vi "Leakage_SMU_PPMU_Test.vi"(0 "Semiconductor Module Context":T4, 5 "Pin Force":T2, 7 "Pins Meas":T2[](array[typedef]), 9 "DCPower_Parameters":T1={"Output"=enum."DC Voltage", "Current_range"=0.0, "Current"=0.0, "Voltage_range"=0.0, "Voltage"=0.0, "Aperture_time"=0.0, "Source Delay"=0.0, "Sense"=1008} {"Source Delay" format="%.6p"; "Sense" items=["Local"=1008, "Remote"=1009]; "Aperture_time" format="%.6p"; "Current_range" format="%.6p"; "Current" format="%.6p"; "Voltage_range" format="%.6p"; "Voltage" format="%.6p"}, 11 "PPMU_Parameters":T3, 12 "Settling (s)":dbl format="%#_6p") -> (15 "error out":errorcluster)   [LabVIEW 2023, in "Leakage.lvlib"]
doc: "Leakage test by forcing one pin with SMU and measuring current with PPMU channels"
uses:
  Leakage.lvlib
  <vilib>/NI_TestStand_SemiconductorModule/NI_TestStand_Semiconductor_Module.lvlibp/PinMap/General/SemiconductorModuleContext.ctl
  <vilib>/NI_TestStand_SemiconductorModule/NI_TestStand_Semiconductor_Module.lvlibp/PinMap/TagProvider/TSM_Pin.ctl
  ResourceHandling/TypeDefs/RH_PPMU_Parameters.ctl
  ResourceHandling/TypeDefs/RH_DCPower_Parameters.ctl
  <instrlib>/niDigital/niDigital.llb/niDigital Output Function.ctl
  <instrlib>/niDigital/niDigital.llb/niDigital Measurement Type.ctl
  <vilib>/NI_TestStand_SemiconductorModule/NI_TestStand_Semiconductor_Module.lvlibp/PinMap/Digital Pattern/SingleSessionPinQueryContext/DigitalPatternSingleSessionPinQueryContext.lvclass
  C:/Program Files/National Instruments/LabVIEW 2023/vi.lib/NI_TestStand_SemiconductorModule/NI_TestStand_Semiconductor_Module.lvlibp/PinMap/PinQueryContext/PinQueryContext.lvclass
  <vilib>/NI_TestStand_SemiconductorModule/NI_TestStand_Semiconductor_Module.lvlibp/PinMap/Digital Pattern/PinsToNIDigitalPatternSession.vi
  <vilib>/NI_TestStand_SemiconductorModule/NI_TestStand_Semiconductor_Module.lvlibp/PinMap/DC Power/PinToNIDCPowerSessions.vi
  <vilib>/NI_TestStand_SemiconductorModule/NI_TestStand_Semiconductor_Module.lvlibp/PinMap/General/Publish/PublishDataDouble1D.vi
  <vilib>/NI_TestStand_SemiconductorModule/NI_TestStand_Semiconductor_Module.lvlibp
  ResourceHandling/ResourceHandling.lvlib
  C:/Program Files/National Instruments/LabVIEW 2023/vi.lib/NI_TestStand_SemiconductorModule/NI_TestStand_Semiconductor_Module.lvlibp/PinMap/PinQueryContext/MultiplePinSingleSessionQueryContext/MultiplePinSingleSessionQueryContext.lvclass
  C:/Program Files/National Instruments/LabVIEW 2023/vi.lib/NI_TestStand_SemiconductorModule/NI_TestStand_Semiconductor_Module.lvlibp/PinMap/Digital Pattern/SingleSessionPinQueryContext/DigitalPatternSingleSessionPinQueryContext.lvclass
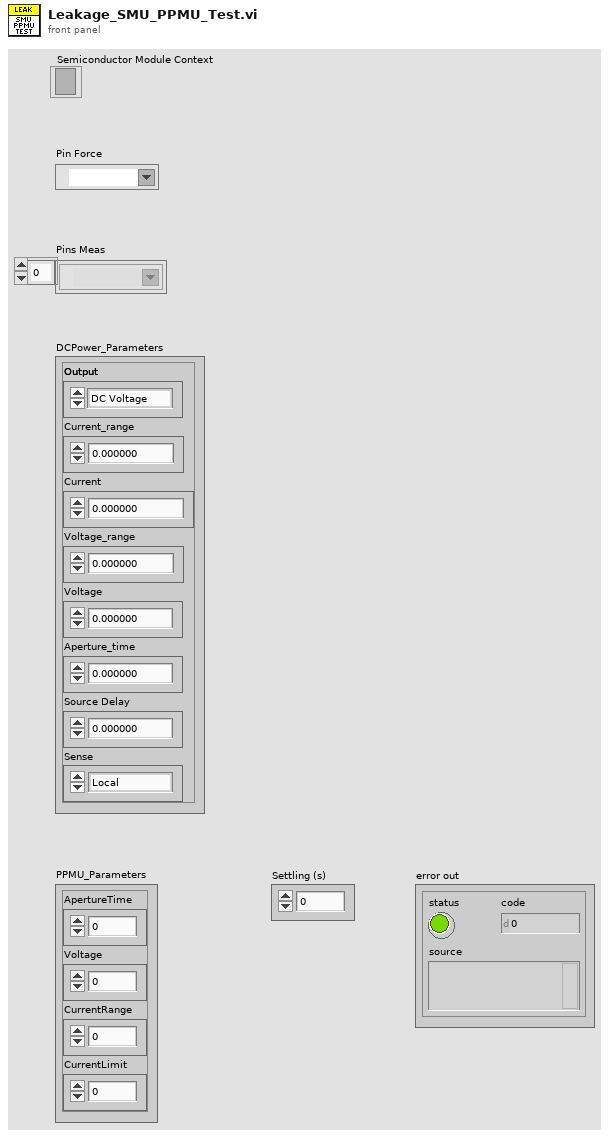
[diagram p1: front panel]
types:
  T1 = typedef "ResourceHandling.lvlib/RH_DCPower_Parameters.ctl" = cluster{"Output":enum16{"DC Voltage", "DC Current"}, "Current_range":dbl, "Current":dbl, "Voltage_range":dbl, "Voltage":dbl, "Aperture_time":dbl, "Source Delay":dbl, "Sense":i32}
  T2 = typedef "NI_TestStand_Semiconductor_Module.lvlibp/TSM_Pin.ctl" = tag
  T3 = typedef "ResourceHandling.lvlib/RH_PPMU_Parameters.ctl" = cluster{"ApertureTime":dbl, "Voltage":dbl, "CurrentRange":dbl, "CurrentLimit":dbl}
  T4 = typedef "NI_TestStand_Semiconductor_Module.lvlibp/SemiconductorModuleContext.ctl" = refnum<k7>
  T5 = typedef "niDigital Measurement Type.ctl" = i32
  T6 = typedef "niDigital Output Function.ctl" = i32
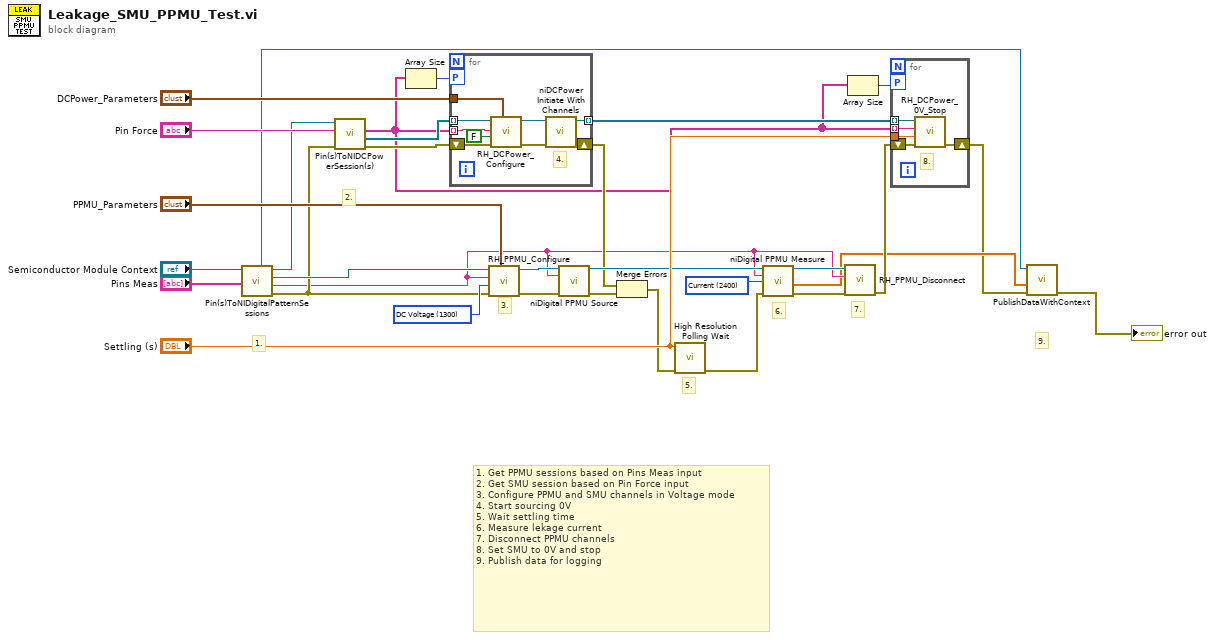
[diagram p0: block diagram]
diagram:
  w21 = T5 2400 items=["Voltage"=2401, "Current"=2400] ("measurement type")
  w26 = T6 1300 items=["DC Voltage"=1300, "DC Current"=1301] ("output function")
  # "9."
  # "7."
  # "6."
  # "5."
  # "3."
  # "2."
  # "1."
  # "1. Get PPMU sessions based on Pins Meas input\n2. Get SMU session based on Pin Force input\n3. Configure PPMU and SMU channels in Voltage mode\n4. Start sourcing 0V\n5. Wait settling time\n6. Measure lekage current\n7. Disconnect PPMU channels\n8. Set SMU to 0V and stop\n9. Publish data for logging"
  n1 = call-poly <vilib>:"Pin(s)ToNIDigitalPatternSessions.vi"("Pins"="Pins Meas", "Semiconductor Module Context"="Semiconductor Module Context") -> ("error out"=w16:errorcluster, "Channel List"=w11:string, "Instrument Session"=w27:refnum<k15>, "Semiconductor Module Context Out"=w17:T4, "Pin Query Context"=w5:refnum<class "DigitalPatternSingleSessionPinQueryContext.lvclass">)  [unwired: 4 in, 1 out]
  n2 = call-poly <vilib>:"Pin(s)ToNIDCPowerSession(s).vi"("error in (no error)"=w16, "Pin"="Pin Force", "Semiconductor Module Context"=w17) -> ("error out"=w15:errorcluster, "Instrument Sessions"=w4:refnum<k15>[], "Channel Strings"=w1:string[])  [unwired: 4 in, 2 out]
  n3 = Array Size(array=w1) -> (size(s)=w3:i32)
  n4 = for {
    tunnel: "DCPower_Parameters" -> [w41]
    tunnel: [w35] -> w9 mode=indexing
    shift-right: [w36] -> w13
    shift-left: w15 -> [w40]
    workers-P: w3 -> [_]
    tunnel: w4 -> [w34] mode=indexing
    tunnel: w1 -> [w33] mode=indexing
    # "4."
    n5 = call "RH_DCPower_Configure.vi"("DCPower_Parameters"=w41, "error in (no error)"=w40, "trigger out?"=FALSE, "channel name"=w33, "DCPower Session In"=w34) -> ("error out"=w37:errorcluster, "DCPower Session Out"=w38:refnum<k15>)  [unwired: 5 in]
    n6 = call <instrlib>:"niDCPower Initiate With Channels.vi"("error in (no error)"=w37, "instrument handle"=w38) -> ("error out"=w36:errorcluster, "instrument handle out"=w35:refnum<k15>)  [unwired: 8 in]
  }
  n7 = call "RH_PPMU_Configure.vi"("Digital_Parameters"="PPMU_Parameters", "error in"=w16, "output function"=w26, "channel list"=w11, "PPMU Session In"=w27) -> ("error out"=w24:errorcluster, "PPMU Session Out"=w25:refnum<k15>)  [unwired: 5 in]
  n8 = call <instrlib>:"niDigital PPMU Source.vi"("instrument handle"=w25, "channel list"=w11, "error in"=w24) -> ("instrument handle out"=w23:refnum<k15>, "error out"=w14:errorcluster)  [unwired: 11 in]
  n9 = Merge Errors(w13, w14) -> (w12:errorcluster)
  n10 = call <vilib>:"High Resolution Polling Wait.vi"("error in (no error)"=w12, "seconds to wait"="Settling (s)") -> ("error out"=w22:errorcluster)  [unwired: 9 in]
  n11 = call <instrlib>:"niDigital PPMU Measure.vi"("instrument handle"=w23, "channel list"=w11, "measurement type"=w21, "error in"=w22) -> ("instrument handle out"=w19:refnum<k15>, "measurements"=w7:dbl[], "error out"=w20:errorcluster)  [unwired: 9 in]
  n12 = call "RH_PPMU_Disconnect.vi"("error in"=w20, "channel list"=w11, "PPMU Session In"=w19) -> ("error out"=w10:errorcluster)  [unwired: 7 in, 1 out]
  n13 = Array Size(array=w1) -> (size(s)=w2:i32)
  n14 = for {
    tunnel: "Settling (s)" -> [w46]
    tunnel: w9 -> [w44] mode=indexing
    shift-right: [w43] -> w6
    shift-left: w10 -> [w45]
    workers-P: w2 -> [_]
    tunnel: w1 -> [w42] mode=indexing
    # "8."
    n15 = call "RH_DCPower_0V_Stop.vi"("error in (no error)"=w45, "Settling (s)"=w46, "Channel List"=w42, "DCPower Session In"=w44) -> ("error out"=w43:errorcluster)  [unwired: 6 in, 1 out]
  }
  n16 = call-poly <vilib>:"PublishDataWithContext.vi"("error in (no error)"=w6, "Data In"=w7, "Pin Query Context"=w5) -> ("error out"=→"error out":errorcluster)  [unwired: 7 in, 1 out]
